vi "PC_accumulate_waveform.vi"(8 "error in":errorcluster, 10 "Time to\n accumulate":dbl, 11 "Waveform":waveform(dbl)) -> (0 "error out":errorcluster, 3 "waveform out":waveform(dbl))   [LabVIEW 2020]
uses:
  <vilib>/Waveform/WDTOps.llb/WDT Append Waveforms DBL.vi
  <vilib>/Waveform/WDTOps.llb/WDT Get Waveform Subset DBL.vi
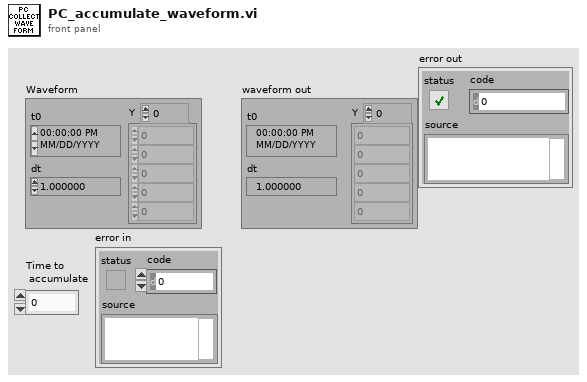
[diagram p1: front panel]
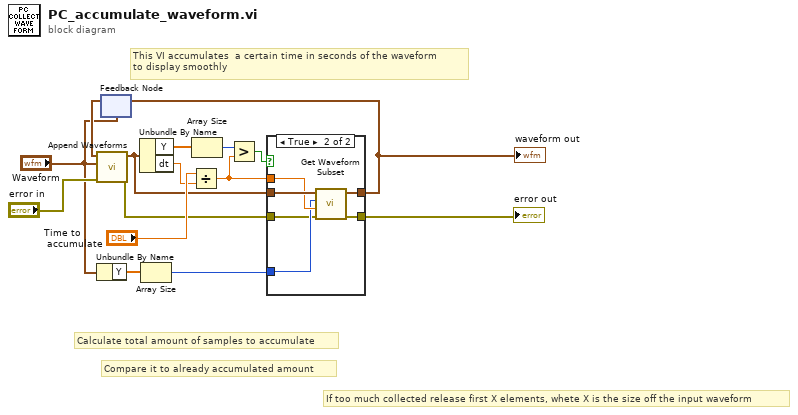
[diagram p0: block diagram]
diagram:
  # "If too much collected release first X elements, whete X is the size off the input waveform"
  # "Compare it to already accumulated amount"
  # "Calculate total amount of samples to accumulate"
  # "This VI accumulates  a certain time in seconds of the waveform \nto display smoothly"
  n1 = Unbundle By Name("Waveform") -> ("Y"=w12:dbl[])
  n2 = feedback #1("Waveform") -> (w13:waveform(dbl))
  n3 = call-poly <vilib>:"Append Waveforms.vi"("error in (no error)"="error in", "waveform B"="Waveform", "waveform A"=w13) -> ("error out"=w3:errorcluster, "waveform out"=w7:waveform(dbl))  [unwired: 7 in]
  n4 = Unbundle By Name(w7) -> ("Y"=w9:dbl[], "dt"=w6:dbl)
  n5 = Array Size(array=w12) -> (size(s)=w11:i32)
  n6 = Divide(x="Time to\n accumulate", y=w6) -> (x/y=w10:dbl)
  n7 = Array Size(array=w9) -> (size(s)=w5:i32)
  n8 = Greater?(x=w5, y=w10) -> (0:w14:bool)
  n9 = case shown="True" w14 {
    tunnel: w7 -> [w17 w23]
    tunnel: [w17 w22] -> w15
    tunnel: w10 -> [_ w21]
    tunnel: w11 -> [_ w20]
    tunnel: w3 -> [w16 w19]
    tunnel: [w16 w18] -> w2
    frame False {
    }
    frame True {
      n10 = call-poly <vilib>:"Get Waveform Subset.vi"("error in (no error)"=w19, "duration"=w21, "start samples/time"=w20, "waveform in"=w23) -> ("error out"=w18:errorcluster, "waveform out"=w22:waveform(dbl))  [unwired: 2 in, 2 out]
    }
  }
  "waveform out" <- w15
  "error out" <- w2
  n11 = feedback-in #1(w15) -> ()
